vi "Read High Level Config Settings.vi"(8 "error in (no error)":errorcluster, 11 "Web FP In":refnum<class "Web Front Panel.lvclass">) -> (0 "error out":errorcluster, 2 "High Level Config Settings":T1, 3 "Web FP Out":refnum<class "Web Front Panel.lvclass">)   [LabVIEW 2015, in "Front Panel Publisher.lvlib" / "Web Front Panel.lvclass"]
uses:
  Web Front Panel.lvclass
  Controls/High Level Config Settings.ctl
  Web Front Panel.lvclass/Web Front Panel.ctl
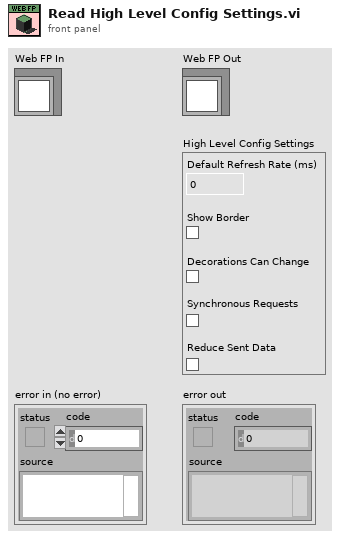
[diagram p1: front panel]
types:
  T1 = typedef "Front Panel Publisher.lvlib/Web Front Panel.lvclass/High Level Config Settings.ctl" = cluster{"Default Refresh Rate (ms)":i32, "Show Border":bool, "Decorations Can Change":bool, "Synchronous Requests":bool, "Reduce Sent Data":bool}
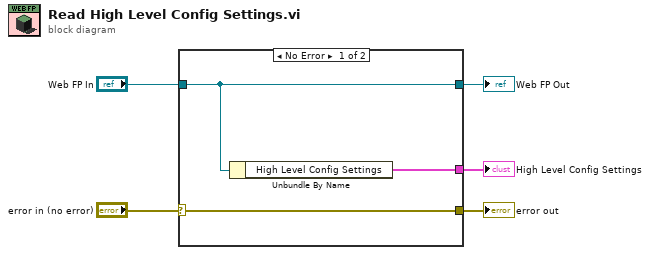
[diagram p0: block diagram]
diagram:
  n1 = case shown="No Error" "error in (no error)" {
    selector: "error in (no error)" -> [w8 w9]
    tunnel: [w8 w9] -> w4
    tunnel: [w7 w10] -> w2
    tunnel: "Web FP In" -> [w7 w10]
    tunnel: [w6 _] -> w1
    frame No Error {
      n2 = Unbundle By Name(w7) -> ("High Level Config Settings"=w6:T1)
    }
    frame Error {
    }
  }
  "error out" <- w4
  "Web FP Out" <- w2
  "High Level Config Settings" <- w1
